vi "Set Error.vi"(8 "error in (no error)":errorcluster, 10 "Message":string, 11 "Code":i32) -> (0 "error out":errorcluster)   [LabVIEW 2016, in "Scan Engine Custom Device.lvlib"]
uses:
  Scan Engine Custom Device.lvlib
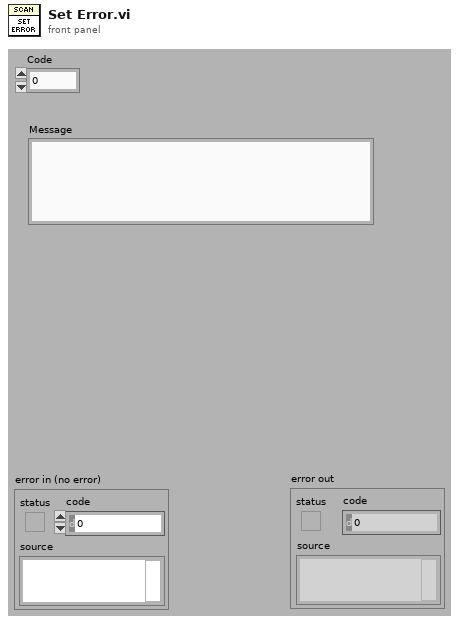
[diagram p1: front panel]
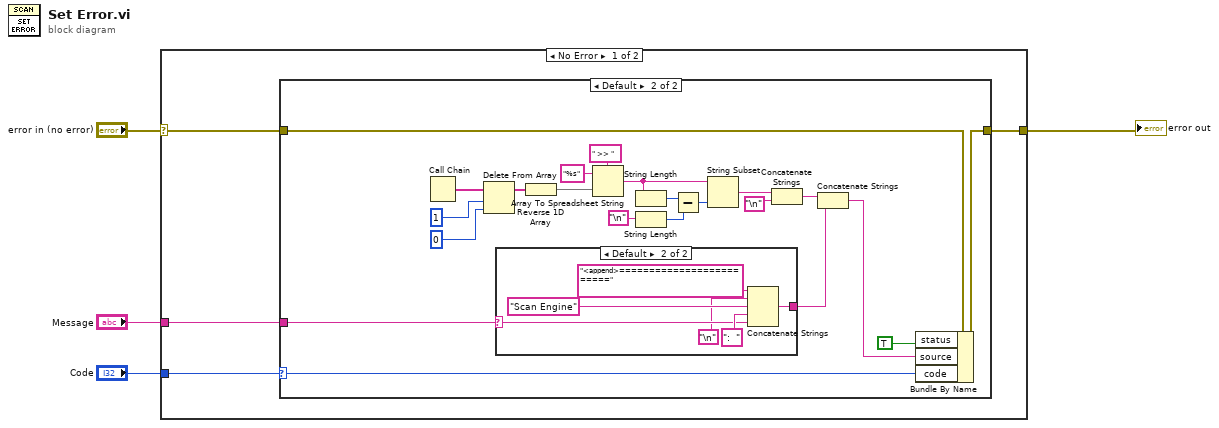
[diagram p0: block diagram]
diagram:
  n1 = case shown="No Error" "error in (no error)" {
    selector: "error in (no error)" -> [w7 w39]
    tunnel: [w8 w39] -> w1
    tunnel: "Code" -> [w6 _]
    tunnel: "Message" -> [w5 _]
    frame No Error {
      n2 = case shown="Default" w6 {
        selector: w6 -> [_ w10]
        tunnel: [w9 w31] -> w8
        tunnel: w7 -> [w9 w12]
        tunnel: w5 -> [_ w11]
        frame 0 {
        }
        frame Default {
          n3 = Call Chain() -> (call chain=w22:string[])
          n4 = Delete From Array(array=w22, length=1 ("CallChainLvl"), index=0) -> (array with subset deleted=w18:string[])  [unwired: 1 out]
          n5 = case shown="Default" w11 {
            selector: w11 -> [w32 w35]
            tunnel: [w32 w36] -> w26
            frame "" {
            }
            frame Default {
              n6 = Concatenate Strings("<append>=========================", "\n", "Scan Engine" ("VeriStand"), ":  " ("string"), w35) -> (w36:string)
            }
          }
          n7 = Reverse 1D Array(array=w18) -> (reversed array=w19:string[])
          n8 = Array To Spreadsheet String(delimiter (Tab)=" >> ", array=w19, 3:"%s" ("format string")) -> (spreadsheet string=w17:string)
          n9 = String Length(string=w17) -> (length=w20:i32)
          n10 = String Length(string="\n") -> (length=w15:i32)
          n11 = Subtract(x=w20, y=w15) -> (x-y=w21:i32)
          n12 = String Subset(string=w17, length (rest)=w21) -> (substring=w27:string)  [unwired: 1 out]
          n13 = Concatenate Strings(w27, "\n") -> (w28:string)
          n14 = Concatenate Strings(w28, w26) -> (w29:string)
          n15 = Bundle By Name(cluster=w12, "status"=TRUE, "source"=w29, "code"=w10) -> (w31:errorcluster)
        }
      }
    }
    frame Error {
      # "Cluster already contains error"
    }
  }
  "error out" <- w1
